vi "Cluster_Left Cell String.vi"(7 "Action":T1=enum."Wire Properties", 11 "Cluster Element Data":T2) -> (2 "Disable":bool, 3 "Left Cell String":string)   [LabVIEW 2023]
doc: "Generate left cell string depending on dialog/action and whether cluster element is labeled."
uses:
  Cluster Element Description.ctl
  controls/action enum.ctl
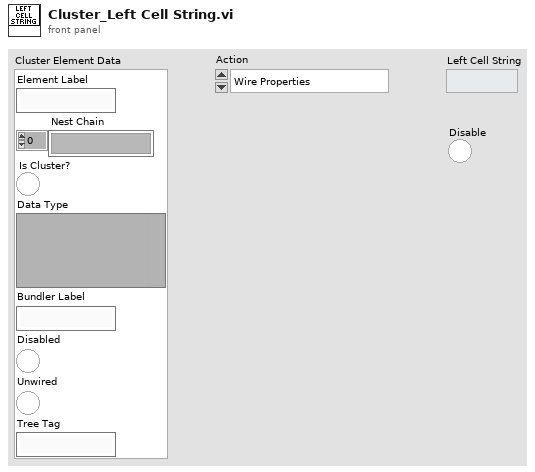
[diagram p1: front panel]
types:
  T1 = typedef "action enum.ctl" = enum16{"[NONE]", "APP_SEPARATOR", "Wire Bundle", "Wire Unbundle", "Terminal Unbundle", "Terminal Bundle", "Bundler Move Up", "Bundler Move Down", "Bundler Insert", "Bundler Remove", "Bundler Remove Unwired", "Bundler Reorder", "In Place Insert", "In Place Remove", "In Place Remove Unwired", "In Place Reorder", "Wire Properties", "Wire Method", "Terminal Properties", "Terminal Method", "Property Move Up", "Property Move Down", "Properties Insert", "Properties Remove", "Properties Remove Unwired", "Properties Reorder", "Method Change", "Class For Constant", "Class For Control", "Class For Node", "Class Name to Clipboard"}
  T2 = typedef "Cluster Element Description.ctl" = cluster{"Element Label":string, "Nest Chain":string[], "Is Cluster?":bool, "Data Type":variant, "Bundler Label":string, "Disabled":bool, "Unwired":bool, "Tree Tag":string}
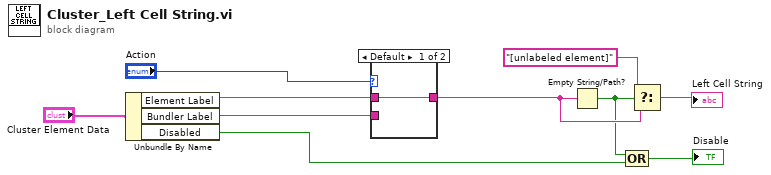
[diagram p0: block diagram]
diagram:
  n1 = Unbundle By Name("Cluster Element Data") -> ("Element Label"=w9:string, "Bundler Label"=w8:string, "Disabled"=w2:bool)
  n2 = case shown="Default" "Action" {
    tunnel: [w11 w12] -> w6
    tunnel: w9 -> [w11 _]
    tunnel: w8 -> [_ w12]
    frame Default {
    }
    frame "Bundler Remove".."Bundler Reorder", "In Place Remove".."In Place Reorder" {
    }
  }
  n3 = Empty String/Path?(string/path=w6) -> (empty?=w3:bool)
  n4 = Compound Arithmetic op=OR(w3, w2) -> (→"Disable":bool)
  n5 = Select(t="[unlabeled element]", s=w3, f=w6) -> (s? t:f=→"Left Cell String":string)
